vi "__Alicat SD_ReadFlows.vi"(6 "Nodos":i32=3, 8 "error in":errorcluster, 10 "aDispositivos":T1=[["A", "SI", "398519", "N2", "100", "SLPM", "0.00", "0.00"], ["B", "SI", "398518", "N2", "100", "SLPM", "0.00", "0.00"], ["C", "SI", "428058", "Air", "100", "SLPM", "0.00", "0.00"], ["D", "NO", "--------", "------", "------", "------", "0.00", "0.00"]] caption="Alicats in", 11 "COMMS":T2={"Alicats"="COM6", "Alic"=TRUE, "eValve"="ASRL6::INSTR", "eval"=FALSE, "Eurotherm"="ASRL6::INSTR", "euro"=FALSE, "Cell GAS"="ASRL6::INSTR", "cgas"=FALSE, "Cell H2S"="ASRL6::INSTR", "ch2s"=FALSE}) -> (0 "error out":errorcluster, 1 "ParsedReadingArray":T3[](array[typedef]) {"Total" format="%.2f"; "SetPoint" format="%.2f"; "Mass" format="%.2f"; "Volumetric" format="%.2f"; "Temperature" format="%.2f"; "Pressure" format="%.2f"}, 2 "aDispositivos 2":T1=[["A", "NO", "aM0000013", "Air", "100", "ln/mn", "0.1", "0.11"], ["B", "NO", "aM0000014", "Air", "100", "ln/mn", "0.2", "0.22"], ["C", "NO", "aM0000015", "Air", "100", "ln/mn", "0.3", "0.33"], ["D", "NO", "aM0000016", "Air", "500", "ln/mn", "0.4", "0.44"]] caption="Alicats out")   [LabVIEW 2017]
uses:
  __Alicat SD_ReadingCluster.ctl
  REACTOR_COMUNICACIONES.ctl
  __s_TablaAlicats.ctl
  __Alicat SD_Hardware_Module.ctl
  REACTOR_GLOBALES.vi
panel:
  out "ID(NODO)":string[](array[string])
  out "CONECTADO":bool[](array[boolean])
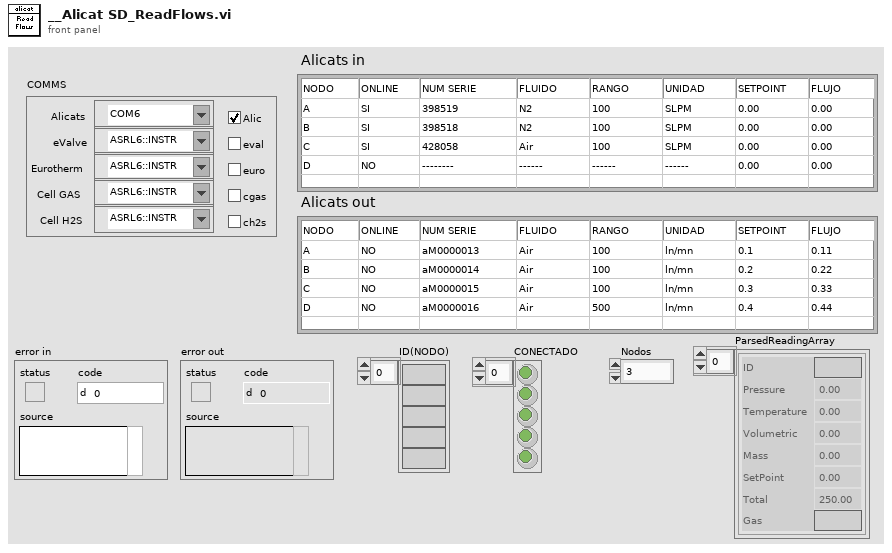
[diagram p1: front panel]
types:
  T1 = typedef "__s_TablaAlicats.ctl" = string[][]
  T2 = typedef "REACTOR_COMUNICACIONES.ctl" = cluster{"Alicats":refnum<visa-resource-name>, "Alic":bool, "eValve":refnum<visa-resource-name>, "eval":bool, "Eurotherm":refnum<visa-resource-name>, "euro":bool, "Cell GAS":refnum<visa-resource-name>, "cgas":bool, "Cell H2S":refnum<visa-resource-name>, "ch2s":bool}
  T3 = typedef "__Alicat SD_ReadingCluster.ctl" = cluster{"ID":string, "Pressure":sgl, "Temperature":sgl, "Volumetric":sgl, "Mass":sgl, "SetPoint":sgl, "Gas":string, "Total":sgl}
  T4 = typedef "__Alicat SD_Hardware_Module.ctl" = enum16{"Initialize", "Send Setpoint", "Read Data", "Change Address", "Shutdown"}
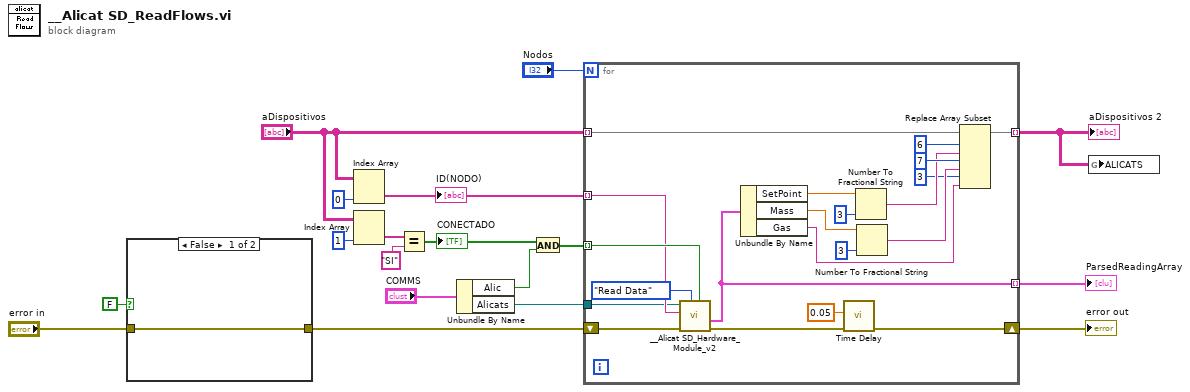
[diagram p0: block diagram]
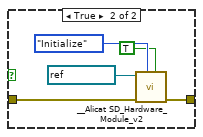
[diagram p2: hidden frame]
diagram:
  n1 = case shown="False" FALSE {
    tunnel: "error in" -> [w19 w24]
    tunnel: [w19 w23] -> w11
    frame False {
    }
    frame True {
      n2 = call "__Alicat SD_Hardware_Module_v2.vi"("Used ?"=TRUE, "Command"=__Alicat_SD_Hardware_Module."Initialize", "error in (no error)"=w24, "VISA resource name"=refnum<visa-resource-name> "COM26") -> ("error out"=w23:errorcluster)  [unwired: 4 in, 3 out]
    }
  }
  n3 = Index Array(array="aDispositivos", index (col)=0 ("disabled index (col)")) -> (element=w14:string[])  [unwired: 1 in]
  "ID(NODO)" <- w14
  n4 = Index Array(array="aDispositivos", index (col)=1 ("disabled index (col)")) -> (element=w17:string[])  [unwired: 1 in]
  n5 = Equal?(x=w17, y="SI") -> (x = y?=w8:bool[])
  "CONECTADO" <- w8
  n6 = Unbundle By Name("COMMS") -> ("Alic"=w7:bool, "Alicats"=w1:refnum<visa-resource-name>)
  n7 = And(x=w8, y=w7) -> (x .and. y?=w9:bool[])
  n8 = for {
    N: "Nodos" -> [_]
    shift-right: [w39] -> w13
    shift-left: w11 -> [w45]
    tunnel: w9 -> [w43] mode=indexing
    tunnel: w14 -> [w42] mode=indexing
    tunnel: [w38] -> w6 mode=indexing
    tunnel: "aDispositivos" -> [w33] mode=indexing
    tunnel: [w32] -> w2 mode=indexing
    tunnel: w1 -> [w25]
    n9 = call "__Alicat SD_Hardware_Module_v2.vi"("Used ?"=w43, "Command"=__Alicat_SD_Hardware_Module."Read Data", "error in (no error)"=w45, "Address"=w42, "VISA resource name"=w25) -> ("error out"=w40:errorcluster, "ParsedReading"=w38:T3)  [unwired: 3 in, 2 out]
    n10 = Unbundle By Name(w38) -> ("SetPoint"=w37:sgl, "Mass"=w36:sgl, "Gas"=w28:string)
    n11 = call "Time Delay"("error in (no error)"=w40, "Delay Time (s)"=0.05) -> ("error out"=w39:errorcluster)  [unwired: 9 in]
    n12 = Number To Fractional String(number=w37, precision (6)=i16 3) -> (F-format string=w31:string)  [unwired: 2 in]
    n13 = Number To Fractional String(number=w36, precision (6)=i16 3) -> (F-format string=w30:string)  [unwired: 2 in]
    n14 = Replace Array Subset(array=w33, new element #1=w31, index #1=6 ("index"), new element #2=w30, index #2=7 ("index"), new element #3=w28, index #3=3 ("index")) -> (w32:string[])
  }
  "error out" <- w13
  "ParsedReadingArray" <- w6
  "aDispositivos 2" <- w2
  n15 = global write "REACTOR_GLOBALES.vi" "ALICATS"(w2) -> ()
